vi "slscswitch Get Relay Position.vi"(8 "error in (no error)":errorcluster, 10 "relay name":string, 11 "SLSC Switch in":refnum<class "SLSC Switch.lvclass">) -> (0 "error out":errorcluster, 2 "position":T1=10 items=["Open"=10, "Closed"=11], 3 "SLSC Switch out":refnum<class "SLSC Switch.lvclass">)   [LabVIEW 2015, in "SLSC Switch.lvclass"]
uses:
  SLSC Switch.lvclass
  Route Manager/Position.ctl
  SLSC Switch.lvclass/SLSC Switch.ctl
  Route Manager/Route Manager.lvclass
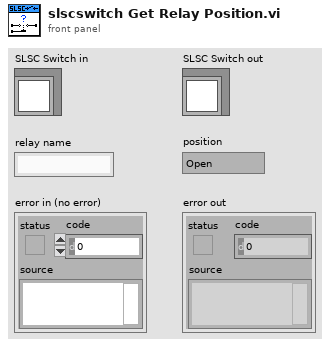
[diagram p1: front panel]
types:
  T1 = typedef "Route Manager.lvclass/Position.ctl" = i32
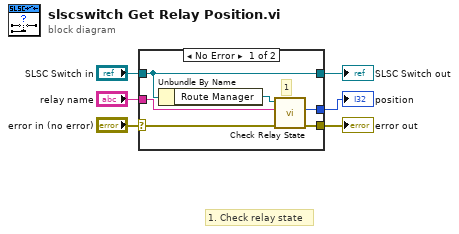
[diagram p0: block diagram]
diagram:
  # "1. Check relay state"
  n1 = case shown="No Error" "error in (no error)" {
    selector: "error in (no error)" -> [w8 w14]
    tunnel: [w7 w14] -> w5
    tunnel: [w11 w13] -> w3
    tunnel: "SLSC Switch in" -> [w11 w13]
    tunnel: "relay name" -> [w12 _]
    tunnel: [w9 _] -> w1
    frame No Error {
      # "1"
      n2 = Unbundle By Name(w11) -> ("Route Manager"=w10:refnum<class "Route Manager.lvclass">)
      n3 = call "Check Relay State.vi"("error in (no error)"=w8, "relay string"=w12, "Route Manager in"=w10) -> ("error out"=w7:errorcluster, "position"=w9:T1)  [unwired: 7 in]
    }
    frame Error {
    }
  }
  "error out" <- w5
  "SLSC Switch out" <- w3
  "position" <- w1
